vi "Subvi_Training_Baseline_통합버전.vi"(4 "Nontarget_Flash_Order":i32[][](array[numeric]), 5 "Target_Flash_Order":i64[](array[numeric]), 6 "samples per channel":i32=25, 7 "Brain_data_source":dbl[][](array[numeric]) caption="EEG_Raw_Data" format="%0.3f", 8 "rate":dbl=500.0 caption="Rate" format="%0.2f", 9 "Experimentation_num":i32=2, 10 "Random_num":i32=9, 11 "Random_Repeat":i32=20) -> (0 "Target_ERP":dbl[][](array[numeric]), 1 "NonTarget":dbl[][](array[numeric]), 2 "Nontarget_ERP":dbl[][](array[numeric]), 3 "Target":dbl[][](array[numeric]))   [LabVIEW 2013]
uses:
  <vilib>/Analysis/3filter.llb/Filter Passband Type.ctl
  <vilib>/Analysis/baseanly.llb/Mean (DBL).vi
  <vilib>/Analysis/3filter.llb/Butterworth Filter (DBL).vi
  <vilib>/Analysis/NI_AALBase.lvlib
  <vilib>/Utility/file.llb/Read From Spreadsheet File (DBL).vi
panel:
  in  "rate 3":dbl=500.0 caption="Rate" format="%0.2f"
  in  "rate 2":dbl=500.0 caption="Rate" format="%0.2f"
  out "Numeric":dbl
  in  "Target_Flash_Order":path=path "C:/Users/Administrator/Desktop/공공복지안전사업연구-노수진/파일럿20130902/전선미1_Training_Test/nontarget_order.xls"
  in  "nontarget order":path=path "C:/Users/Administrator/Desktop/공공복지안전사업연구-노수진/파일럿20130902/전선미1_Training_Test/nontarget_order.xls"
  in  "Raw Data(EEG)":path=path "C:/Users/Administrator/Desktop/공공복지안전사업연구-노수진/파일럿20130902/전선미1_Training_Test/brain.xls"
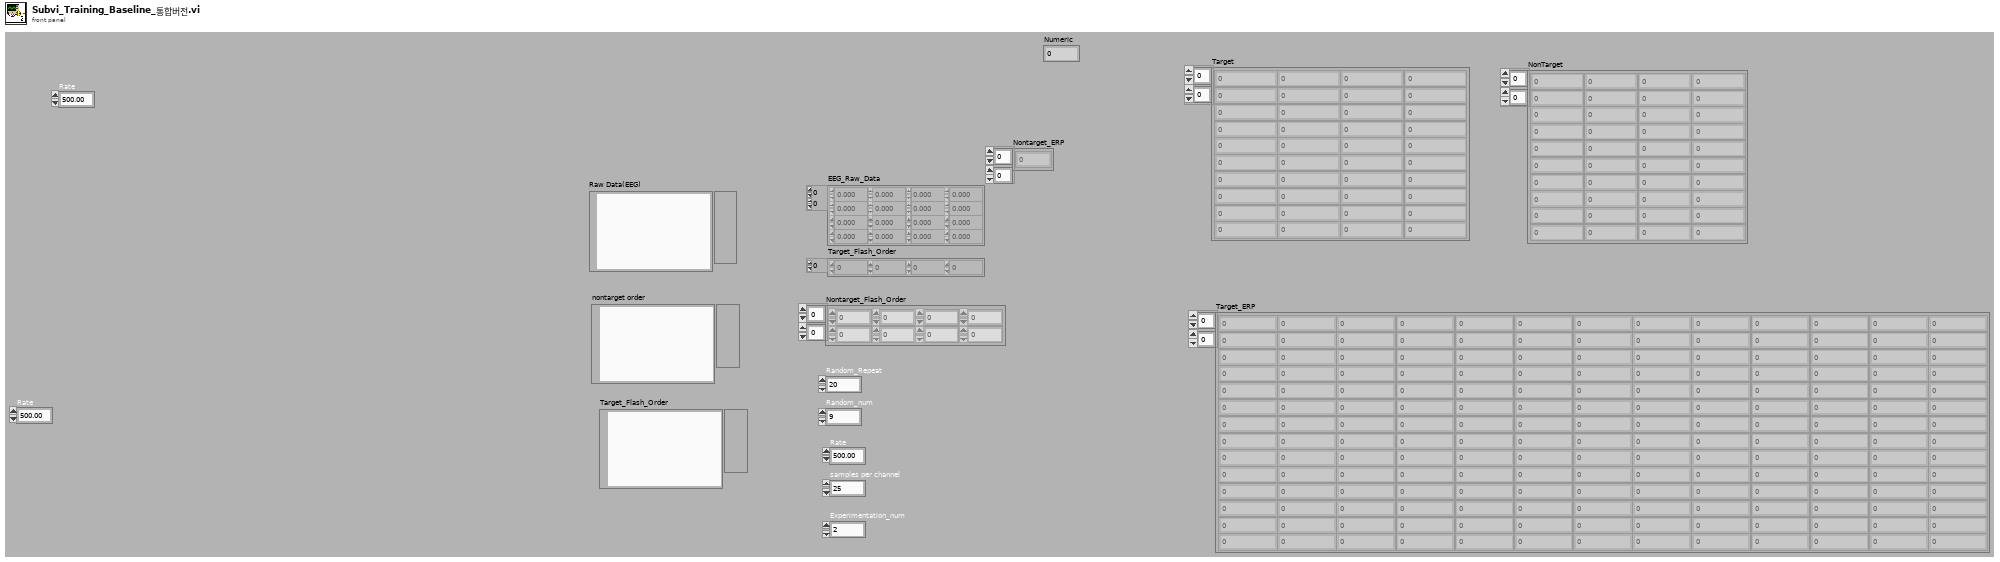
[diagram p1: front panel]
types:
  T1 = typedef "NI_AALBase.lvlib/Filter Passband Type.ctl" = enum32{"Lowpass", "Highpass", "Bandpass", "Bandstop"}
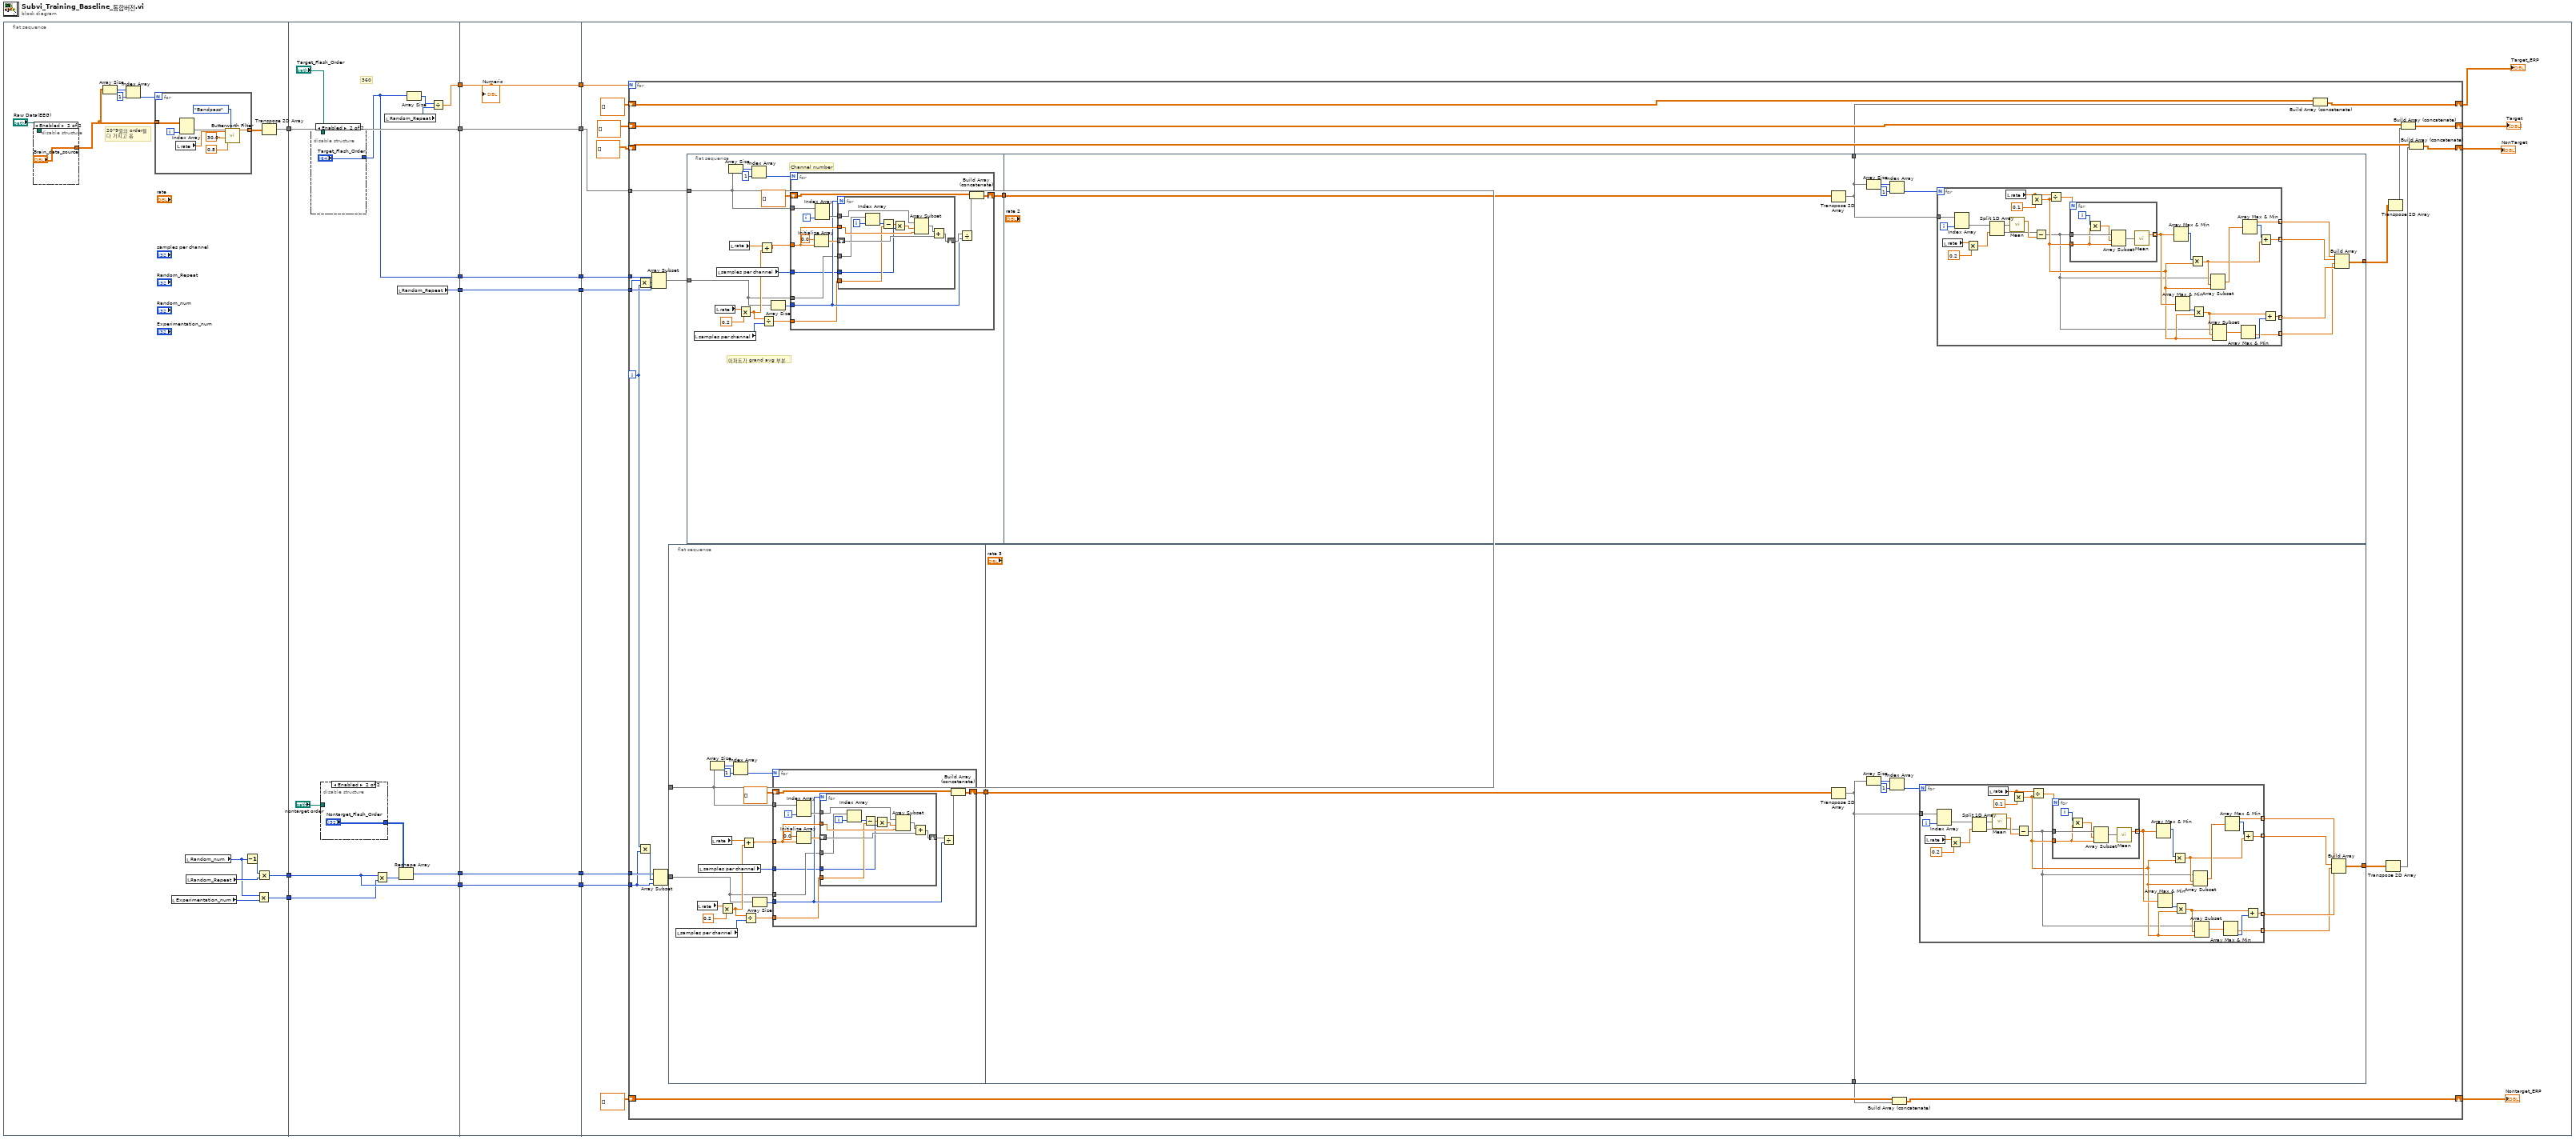
[diagram p0: block diagram]
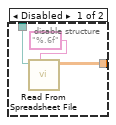
[diagram p2: hidden frame]
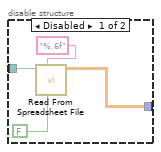
[diagram p3: hidden frame]
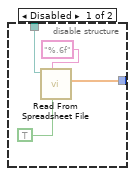
[diagram p4: hidden frame]
diagram:
  n1 = flat-sequence {
    tunnel: [w24] -> w15
    tunnel: [w21] -> w14
    tunnel: [w18] -> w13
    tunnel: w15 -> [w53]
    tunnel: [w53] -> w12
    tunnel: [w50] -> w10
    tunnel: [w42] -> w8
    tunnel: [w49] -> w6
    tunnel: w14 -> [w46]
    tunnel: [w47] -> w4
    tunnel: [w46] -> w2
    tunnel: w13 -> [w45]
    tunnel: w12 -> [w64]
    tunnel: [w64] -> w11
    tunnel: w10 -> [w69]
    tunnel: [w69] -> w9
    tunnel: w8 -> [w68]
    tunnel: [w68] -> w7
    tunnel: w6 -> [w67]
    tunnel: [w67] -> w5
    tunnel: w4 -> [w66]
    tunnel: [w66] -> w3
    tunnel: w2 -> [w65]
    tunnel: [w65] -> w1
    tunnel: w11 -> [w83]
    tunnel: w9 -> [w74]
    tunnel: w7 -> [w82]
    tunnel: w5 -> [w81]
    tunnel: w3 -> [w80]
    tunnel: w1 -> [w79]
    frame #0 {
      # "20*9열의 order를\n다 가지고 옴"
      n2 = disable-structure shown="Enabled" {
        disable-tunnel: [w30 "Brain_data_source"] -> w17
        disable-tunnel: "Raw Data(EEG)" -> [w29 _]
        frame Disabled {
          n3 = call-poly <vilib>:"Read From Spreadsheet File.vi"("format (%.3f)"="%.6f", "file path (dialog if empty)"=w29) -> ("all rows"=w30:dbl[][])  [unwired: 5 in, 4 out]
        }
        frame Enabled {
        }
      }
      n4 = Array Size(array=w17) -> (size(s)=w25:i32[])
      n5 = Index Array(array=w25, index=1) -> (element=w27:i32)
      n6 = for {
        N: w27 -> [_]
        tunnel: w17 -> [w40]
        tunnel: [w36] -> w28 mode=indexing
        i -> [w39]
        n7 = local read "rate"() -> (w33:dbl)
        n8 = Index Array(array=w40, index (col)=w39) -> (element=w38:dbl[])  [unwired: 1 in]
        n9 = call-poly <vilib>:"Butterworth Filter.vi"("filter type"=Filter_Passband_Type."Bandpass", "low cutoff freq: fl"=0.5, "high cutoff freq: fh"=30.0, "sampling freq: fs"=w33, "X"=w38) -> ("Filtered X"=w36:dbl[])  [unwired: 3 in, 1 out]
      }
      n10 = local read "Experimentation_num"() -> (w20:i32)
      n11 = local read "Random_num"() -> (w19:i32)
      n12 = local read "Random_Repeat"() -> (w22:i32)
      n13 = Decrement(x=w19) -> (x-1=w23:i32)
      n14 = Multiply(x=w19, y=w20) -> (x*y=w18:i32)
      n15 = Multiply(x=w23, y=w22) -> (x*y=w21:i32)
      n16 = Transpose 2D Array(2D array=w28) -> (transposed array=w24:dbl[][])
    }
    frame #1 {
      # "360"
      n17 = disable-structure shown="Enabled" {
        disable-tunnel: [w60 "Target_Flash_Order"] -> w42
        disable-tunnel: "Target_Flash_Order" -> [w59 _]
        frame Disabled {
          n18 = call-poly <vilib>:"Read From Spreadsheet File.vi"("transpose (no:F)"=TRUE, "format (%.3f)"="%.6f", "file path (dialog if empty)"=w59) -> ("first row"=w60:dbl[])  [unwired: 4 in, 4 out]
        }
        frame Enabled {
        }
      }
      n19 = disable-structure shown="Enabled" {
        disable-tunnel: "nontarget order" -> [w57 _]
        disable-tunnel: [w55 "Nontarget_Flash_Order"] -> w43
        frame Disabled {
          n20 = call-poly <vilib>:"Read From Spreadsheet File.vi"("transpose (no:F)"=FALSE, "format (%.3f)"="%.6f", "file path (dialog if empty)"=w57) -> ("all rows"=w55:dbl[][])  [unwired: 4 in, 4 out]
        }
        frame Enabled {
        }
      }
      n21 = Multiply(x=w46, y=w45) -> (x*y=w48:i32)
      n22 = local read "Random_Repeat"() -> (w51:i32)
      n23 = local read "Random_Repeat"() -> (w49:i32)
      n24 = Reshape Array(w43, w48) -> (w47:i32[])
      n25 = Array Size(array=w42) -> (size(s)=w52:i32)
      n26 = Divide(x=w52, y=w51) -> (x/y=w50:dbl)
    }
    frame #2 {
      "Numeric" <- w69
    }
    frame #3 {
      n27 = for {
        N: w74 -> [_]
        tunnel: w83 -> [w103]
        tunnel: w82 -> [w109]
        tunnel: w81 -> [w107]
        tunnel: w80 -> [w100]
        tunnel: w79 -> [w98]
        shift-right: [w96] -> w76
        shift-left: dbl[][] [] -> [w97]
        shift-right: [w95] -> w75
        shift-left: dbl[][] [] -> [w94]
        shift-right: [w86] -> w70
        shift-left: dbl[][] [] -> [w84]
        shift-right: [w87] -> w72
        shift-left: dbl[][] [] -> [w89]
        i -> [w101]
        n28 = Multiply(x=w107, y=w101) -> (x*y=w108:i32)
        n29 = Multiply(x=w101, y=w98) -> (x*y=w102:i32)
        n30 = Array Subset(array=w109, index=w108, length=w107) -> (w106:i64[])
        n31 = Array Subset(array=w100, index=w102, length=w98) -> (w99:i32[])
        n32 = flat-sequence {
          tunnel: w103 -> [w112]
          tunnel: w99 -> [w111]
          tunnel: [w110] -> w104
          tunnel: w104 -> [w159]
          tunnel: [w158] -> w91
          tunnel: [w157] -> w88
          frame #0 {
            n33 = local read "samples per channel"() -> (w119:i32)
            n34 = local read "rate"() -> (w121:dbl)
            n35 = local read "samples per channel"() -> (w118:i32)
            n36 = Array Size(array=w112) -> (size(s)=w115:i32[])
            n37 = local read "rate"() -> (w123:dbl)
            n38 = Multiply(x=w121, y=0.2) -> (x*y=w125:dbl)
            n39 = Index Array(array=w115, index=1) -> (element=w117:i32)
            n40 = Add(x=w123, y=w125) -> (x+y=w124:dbl)
            n41 = Divide(x=w125, y=w119) -> (x/y=w122:dbl)
            n42 = Array Size(array=w111) -> (size(s)=w114:i32)
            n43 = for {
              N: w117 -> [_]
              tunnel: w118 -> [w126]
              tunnel: w124 -> [w137]
              shift-right: [w130] -> w110
              shift-left: dbl[][] [] -> [w132]
              tunnel: w114 -> [w131]
              tunnel: w112 -> [w129]
              tunnel: w111 -> [w128]
              tunnel: w122 -> [w127]
              i -> [w139]
              n44 = Initialize Array(0.0 ("element"), w137) -> (w136:dbl[])
              n45 = Index Array(array=w129, index (col)=w139) -> (element=w138:dbl[])  [unwired: 1 in]
              n46 = for {
                N: w131 -> [_]
                tunnel: w138 -> [w151]
                shift-right: [w147] -> w134
                shift-left: w136 -> [w148]
                tunnel: w137 -> [w146]
                tunnel: w128 -> [w144]
                tunnel: w127 -> [w142]
                tunnel: w126 -> [w140]
                i -> [w145]
                n47 = Index Array(array=w144, index=w145) -> (element=w143:i32)
                n48 = Subtract(x=w143, y=w142) -> (x-y=w141:dbl)
                n49 = Multiply(x=w141, y=w140) -> (x*y=w150:dbl)
                n50 = Array Subset(array=w151, index=w150, length=w146) -> (w149:dbl[])
                n51 = Add(x=w149, y=w148) -> (x+y=w147:dbl[])
              }
              n52 = Divide(x=w134, y=w131) -> (x/y=w133:dbl[])
              n53 = Build Array (concatenate)(w132, w133) -> (w130:dbl[][])
            }
          }
          frame #1 {
            n54 = Transpose 2D Array(2D array=w159) -> (transposed array=w157:dbl[][])
            n55 = Array Size(array=w157) -> (size(s)=w161:i32[])
            n56 = Index Array(array=w161, index=1) -> (element=w156:i32)
            n57 = for {
              N: w156 -> [_]
              tunnel: w157 -> [w188]
              tunnel: [w179] -> w155 mode=indexing
              tunnel: [w177] -> w154 mode=indexing
              tunnel: [w171] -> w152 mode=indexing
              tunnel: [w170] -> w153 mode=indexing
              i -> [w169]
              n58 = local read "rate"() -> (w187:dbl)
              n59 = Index Array(array=w188, index (col)=w169) -> (element=w176:dbl[])  [unwired: 1 in]
              n60 = Multiply(x=w187, y=0.2) -> (x*y=w185:dbl)
              n61 = Split 1D Array(array=w176, index=w185) -> (first subarray=w184:dbl[], second subarray=w165:dbl[])
              n62 = local read "rate"() -> (w181:dbl)
              n63 = call-poly <vilib>:"Mean.vi"("X"=w184) -> ("mean"=w183:dbl)  [unwired: 1 out]
              n64 = Multiply(x=w181, y=0.1) -> (x*y=w163:dbl)
              n65 = Subtract(x=w165, y=w183) -> (x-y=w162:dbl[])
              n66 = Divide(x=w181, y=w163) -> (x/y=w180:dbl)
              n67 = for {
                N: w180 -> [_]
                tunnel: w162 -> [w193]
                tunnel: [w194] -> w175 mode=indexing
                tunnel: w163 -> [w191]
                i -> [w190]
                n68 = Multiply(x=w190, y=w191) -> (x*y=w192:dbl)
                n69 = Array Subset(array=w193, index=w192, length=w191) -> (w189:dbl[])
                n70 = call-poly <vilib>:"Mean.vi"("X"=w189) -> ("mean"=w194:dbl)  [unwired: 1 out]
              }
              n71 = Array Max & Min(array=w175) -> (max index (indices)=w168:i32)  [unwired: 3 out]
              n72 = Array Max & Min(array=w175) -> (min index (indices)=w167:i32)  [unwired: 3 out]
              n73 = Multiply(x=w168, y=w163) -> (x*y=w164:dbl)
              n74 = Multiply(x=w167, y=w163) -> (x*y=w173:dbl)
              n75 = Array Subset(array=w162, index=w164, length=w163) -> (w166:dbl[])
              n76 = Array Subset(array=w162, index=w173, length=w163) -> (w174:dbl[])
              n77 = Array Max & Min(array=w174) -> (min value=w171:dbl, min index (indices)=w172:i32)  [unwired: 2 out]
              n78 = Array Max & Min(array=w166) -> (max value=w179:dbl, max index (indices)=w178:i32)  [unwired: 2 out]
              n79 = Add(x=w178, y=w164) -> (x+y=w177:dbl)
              n80 = Add(x=w173, y=w172) -> (x+y=w170:dbl)
            }
            n81 = Build Array(w155, w154, w152, w153) -> (w158:dbl[][])
          }
        }
        n82 = flat-sequence {
          tunnel: w103 -> [w197]
          tunnel: w106 -> [w196]
          tunnel: [w195] -> w105
          tunnel: w105 -> [w244]
          tunnel: [w243] -> w93
          tunnel: [w241] -> w85
          frame #0 {
            # "Channel number"
            # "이파트가 grand avg 부분"
            n83 = local read "samples per channel"() -> (w204:i32)
            n84 = local read "rate"() -> (w206:dbl)
            n85 = local read "samples per channel"() -> (w203:i32)
            n86 = Array Size(array=w197) -> (size(s)=w200:i32[])
            n87 = local read "rate"() -> (w208:dbl)
            n88 = Multiply(x=w206, y=0.2) -> (x*y=w210:dbl)
            n89 = Index Array(array=w200, index=1) -> (element=w202:i32)
            n90 = Add(x=w208, y=w210) -> (x+y=w209:dbl)
            n91 = Divide(x=w210, y=w204) -> (x/y=w207:dbl)
            n92 = Array Size(array=w196) -> (size(s)=w199:i32)
            n93 = for {
              N: w202 -> [_]
              tunnel: w203 -> [w211]
              tunnel: w209 -> [w222]
              shift-right: [w215] -> w195
              shift-left: dbl[][] [] -> [w217]
              tunnel: w199 -> [w216]
              tunnel: w197 -> [w214]
              tunnel: w196 -> [w213]
              tunnel: w207 -> [w212]
              i -> [w224]
              n94 = Initialize Array(0.0 ("element"), w222) -> (w221:dbl[])
              n95 = Index Array(array=w214, index (col)=w224) -> (element=w223:dbl[])  [unwired: 1 in]
              n96 = for {
                N: w216 -> [_]
                tunnel: w223 -> [w236]
                shift-right: [w232] -> w219
                shift-left: w221 -> [w233]
                tunnel: w222 -> [w231]
                tunnel: w213 -> [w229]
                tunnel: w212 -> [w227]
                tunnel: w211 -> [w225]
                i -> [w230]
                n97 = Index Array(array=w229, index=w230) -> (element=w228:i64)
                n98 = Subtract(x=w228, y=w227) -> (x-y=w226:dbl)
                n99 = Multiply(x=w226, y=w225) -> (x*y=w235:dbl)
                n100 = Array Subset(array=w236, index=w235, length=w231) -> (w234:dbl[])
                n101 = Add(x=w234, y=w233) -> (x+y=w232:dbl[])
              }
              n102 = Divide(x=w219, y=w216) -> (x/y=w218:dbl[])
              n103 = Build Array (concatenate)(w217, w218) -> (w215:dbl[][])
            }
          }
          frame #1 {
            n104 = Transpose 2D Array(2D array=w244) -> (transposed array=w241:dbl[][])
            n105 = Array Size(array=w241) -> (size(s)=w246:i32[])
            n106 = Index Array(array=w246, index=1) -> (element=w240:i32)
            n107 = for {
              N: w240 -> [_]
              tunnel: w241 -> [w273]
              tunnel: [w264] -> w242 mode=indexing
              tunnel: [w262] -> w239 mode=indexing
              tunnel: [w256] -> w237 mode=indexing
              tunnel: [w255] -> w238 mode=indexing
              i -> [w254]
              n108 = local read "rate"() -> (w272:dbl)
              n109 = Index Array(array=w273, index (col)=w254) -> (element=w261:dbl[])  [unwired: 1 in]
              n110 = Multiply(x=w272, y=0.2) -> (x*y=w270:dbl)
              n111 = Split 1D Array(array=w261, index=w270) -> (first subarray=w269:dbl[], second subarray=w250:dbl[])
              n112 = local read "rate"() -> (w266:dbl)
              n113 = call-poly <vilib>:"Mean.vi"("X"=w269) -> ("mean"=w268:dbl)  [unwired: 1 out]
              n114 = Multiply(x=w266, y=0.1) -> (x*y=w248:dbl)
              n115 = Subtract(x=w250, y=w268) -> (x-y=w247:dbl[])
              n116 = Divide(x=w266, y=w248) -> (x/y=w265:dbl)
              n117 = for {
                N: w265 -> [_]
                tunnel: w247 -> [w278]
                tunnel: [w279] -> w260 mode=indexing
                tunnel: w248 -> [w276]
                i -> [w275]
                n118 = Multiply(x=w275, y=w276) -> (x*y=w277:dbl)
                n119 = Array Subset(array=w278, index=w277, length=w276) -> (w274:dbl[])
                n120 = call-poly <vilib>:"Mean.vi"("X"=w274) -> ("mean"=w279:dbl)  [unwired: 1 out]
              }
              n121 = Array Max & Min(array=w260) -> (max index (indices)=w253:i32)  [unwired: 3 out]
              n122 = Array Max & Min(array=w260) -> (min index (indices)=w252:i32)  [unwired: 3 out]
              n123 = Multiply(x=w253, y=w248) -> (x*y=w249:dbl)
              n124 = Multiply(x=w252, y=w248) -> (x*y=w258:dbl)
              n125 = Array Subset(array=w247, index=w249, length=w248) -> (w251:dbl[])
              n126 = Array Subset(array=w247, index=w258, length=w248) -> (w259:dbl[])
              n127 = Array Max & Min(array=w259) -> (min value=w256:dbl, min index (indices)=w257:i32)  [unwired: 2 out]
              n128 = Array Max & Min(array=w251) -> (max value=w264:dbl, max index (indices)=w263:i32)  [unwired: 2 out]
              n129 = Add(x=w263, y=w249) -> (x+y=w262:dbl)
              n130 = Add(x=w258, y=w257) -> (x+y=w255:dbl)
            }
            n131 = Build Array(w242, w239, w237, w238) -> (w243:dbl[][])
          }
        }
        n132 = Build Array (concatenate)(w89, w88) -> (w87:dbl[][])
        n133 = Build Array (concatenate)(w84, w85) -> (w86:dbl[][])
        n134 = Transpose 2D Array(2D array=w91) -> (transposed array=w90:dbl[][])
        n135 = Transpose 2D Array(2D array=w93) -> (transposed array=w92:dbl[][])
        n136 = Build Array (concatenate)(w97, w92) -> (w96:dbl[][])
        n137 = Build Array (concatenate)(w94, w90) -> (w95:dbl[][])
      }
      "Target" <- w76
      "NonTarget" <- w75
      "Target_ERP" <- w70
      "Nontarget_ERP" <- w72
    }
  }
